vi "PumpController GetSensorStream Read.vi"(8 "error in":errorcluster, 11 "Call ID in":T2) -> (0 "error out":errorcluster, 1 "Success":bool, 2 "Response Data":T1, 3 "Call ID":T2)   [LabVIEW 2024, in "pumploop_client.lvlib"]
uses:
  pumploop_client.lvlib
  <vilib>/gRPC/LabVIEW gRPC Library/Shared/grpcId.ctl
  RPC Messages/pumploop_Sensors.ctl
  RPC Messages/pumploop_Sensors_Flat.ctl
  aea5dbbb-03a2-479b-ad95-94da4ee1cea9.vi
  <vilib>/gRPC/LabVIEW gRPC Library/Shared/TranslateGrpcError.vi
  <vilib>/gRPC/LabVIEW gRPC Library/Server API/Server/Get Server DLL Path.vi
  <vilib>/Utility/error.llb/Error Cluster From Error Code.vi
  <vilib>/gRPC/LabVIEW gRPC Library/Shared/Wait On Occurrence Wrapper.vi
  <vilib>/gRPC/LabVIEW gRPC Library/grpc-lvsupport-release.lvlib
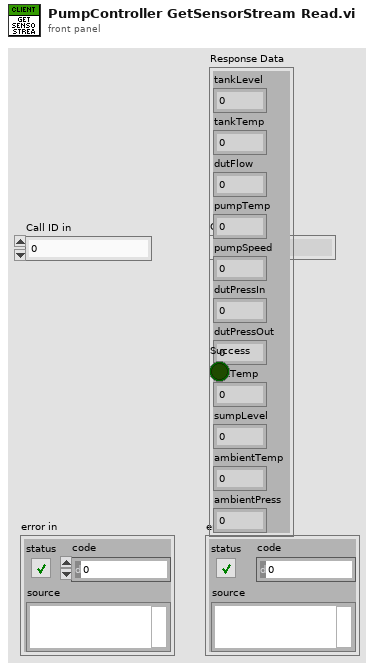
[diagram p1: front panel]
types:
  T1 = typedef "pumploop_client.lvlib/pumploop_Sensors.ctl" = cluster{"tankLevel":sgl, "tankTemp":sgl, "dutFlow":sgl, "pumpTemp":sgl, "pumpSpeed":sgl, "dutPressIn":sgl, "dutPressOut":sgl, "dutTemp":sgl, "sumpLevel":sgl, "ambientTemp":sgl, "ambientPress":sgl}
  T2 = typedef "grpc-lvsupport-release.lvlib/grpcId.ctl" = u64
  T3 = typedef "pumploop_client.lvlib/pumploop_Sensors_Flat.ctl" = cluster{"tankLevel":sgl, "tankTemp":sgl, "dutFlow":sgl, "pumpTemp":sgl, "pumpSpeed":sgl, "dutPressIn":sgl, "dutPressOut":sgl, "dutTemp":sgl, "sumpLevel":sgl, "ambientTemp":sgl, "ambientPress":sgl}
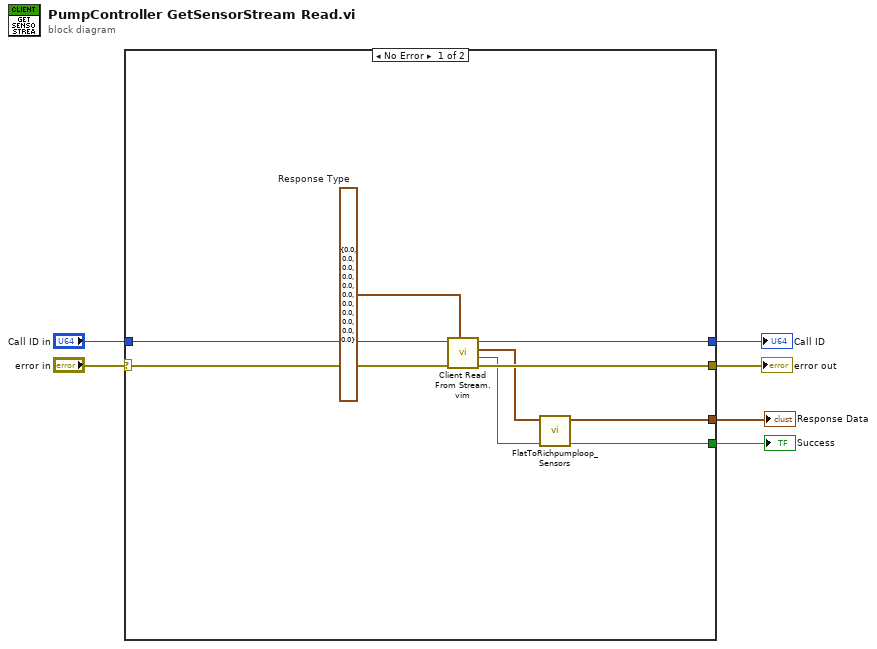
[diagram p0: block diagram]
diagram:
  n1 = case shown="No Error" "error in" {
    selector: "error in" -> [w14 w15]
    tunnel: [w13 w15] -> w5
    tunnel: "Call ID in" -> [w12 w16]
    tunnel: [w10 w16] -> w3
    tunnel: [w7 _] -> w2
    tunnel: [w11 _] -> w1
    frame No Error {
      w9 = T3 {"tankLevel"=0.0, "tankTemp"=0.0, "dutFlow"=0.0, "pumpTemp"=0.0, "pumpSpeed"=0.0, "dutPressIn"=0.0, "dutPressOut"=0.0, "dutTemp"=0.0, "sumpLevel"=0.0, "ambientTemp"=0.0, "ambientPress"=0.0}  # Response Type
      n2 = call "Client Read From Stream.vim"("Response Type"=w9, "error in"=w14, "Call ID in"=w12) -> ("error out"=w13:errorcluster, "Success"=w11:bool, "Response Data"=w8:T3, "Call ID out"=w10:u64)  [unwired: 5 in]
      n3 = call "FlatToRichpumploop_Sensors.vi"("InputCluster"=w8) -> ("OutputCluster"=w7:T1)  [unwired: 10 in]
    }
    frame Error {
    }
  }
  "error out" <- w5
  "Call ID" <- w3
  "Response Data" <- w2
  "Success" <- w1
